vi "Create.vi"(8 "error in (no error)":errorcluster, 9 "Test Method VI Path":path, 10 "Name":string, 11 "Parameterized Test Case":refnum<class "Parameterized Test Case.lvclass">) -> (0 "error out":errorcluster, 3 "Parameter Out":refnum<class "Parameter.lvclass">)   [LabVIEW 2020, in "Parameter.lvclass"]
uses:
  Parameter.lvclass
  <vilib>/Astemes/LUnit/Test Case.lvclass
  Parameterized Test Case/Parameterized Test Case.lvclass
  C:/Program Files (x86)/National Instruments/LabVIEW 2020/vi.lib/Astemes/LUnit/Test Case.lvclass
  C:/Program Files (x86)/National Instruments/LabVIEW 2020/vi.lib/Astemes/LUnit/LUnit Runnable.lvclass
  C:/git/astemes-lunit-parameterized-test/source/Parameterized Test Case/Parameterized Test Case.lvclass
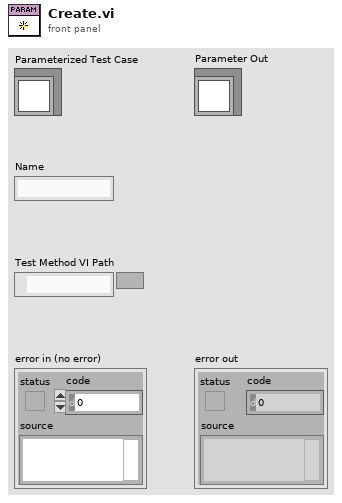
[diagram p1: front panel]
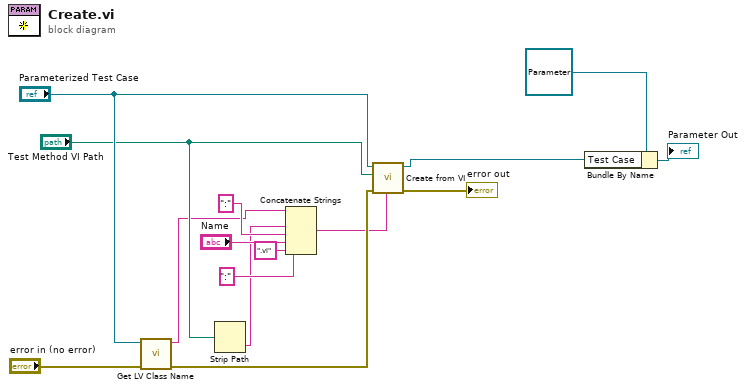
[diagram p0: block diagram]
diagram:
  n1 = call <vilib>:"Get LV Class Name.vi"("error in (no error)"="error in (no error)", "object"="Parameterized Test Case") -> ("error out"=w6:errorcluster, "class name"=w4:string)  [unwired: 8 in]
  n2 = Strip Path(path="Test Method VI Path") -> (name=w2:string)  [unwired: 1 out]
  n3 = Concatenate Strings(w4, ":" ("string"), w2, ":" ("string"), "Name", ".vi" ("string")) -> (w1:string)
  n4 = call <vilib>:"Create from VI.vi"("Test Name"=w1, "error in (no error)"=w6, "Test Method VI Path"="Test Method VI Path", "LUnit Test Case In"="Parameterized Test Case") -> ("error out"=→"error out":errorcluster, "LUnit Test Case Out"=w10:refnum<class "Parameterized Test Case.lvclass">)  [unwired: 6 in]
  n5 = Bundle By Name(cluster=refnum<class "Parameter.lvclass"> refnum ("Parameter"), "Test Case"=w10) -> (→"Parameter Out":refnum<class "Parameter.lvclass">)
